vi "Select Controls 2.vi"(10 "All Controls[]":refnum<vi>[](array[refnum])=[refnum, refnum, refnum, refnum, refnum, refnum, refnum, refnum, refnum]) -> (0 "Create Accessors Folder 2":bool=TRUE, 1 "OK?":bool, 2 "Selection":i32[](array[numeric]), 3 "Operation":T1, 4 "Create Properties 2":bool, 5 "isDynamic?":bool)   [LabVIEW 2018, in "DVR Accessor Library.lvlib"]
uses:
  DVR Accessor Library.lvlib
  TypeDef/Accessor Type.ctl
panel:
  in  "Create Accessors Folder on HD":bool=TRUE
  in  "Type":T1=enum."Read And Write"
  in  "Scope":enum32{"Item 0", "Item 1"}(radio)
  in  "Create Properties":bool=TRUE
  in  "Cancel":bool
  in  "OK":bool
  in  "Data Members":string[](tree)
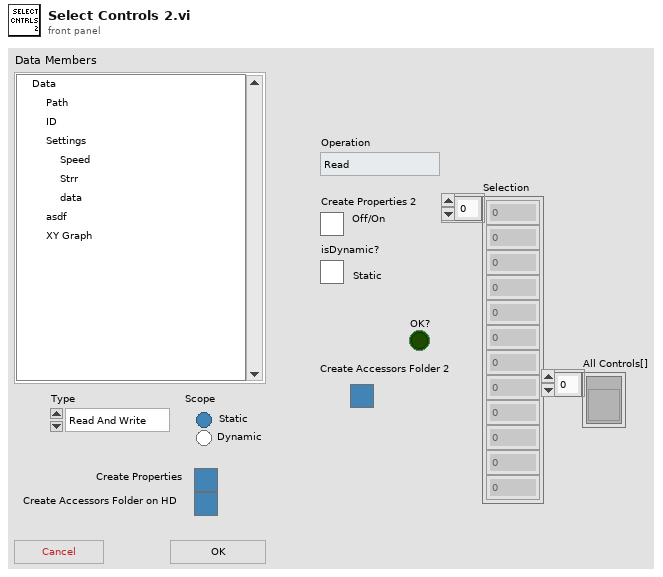
[diagram p1: front panel]
types:
  T1 = typedef "DVR Accessor Library.lvlib/Accessor Type.ctl" = enum16{"Read", "Read And Write", "Write"}
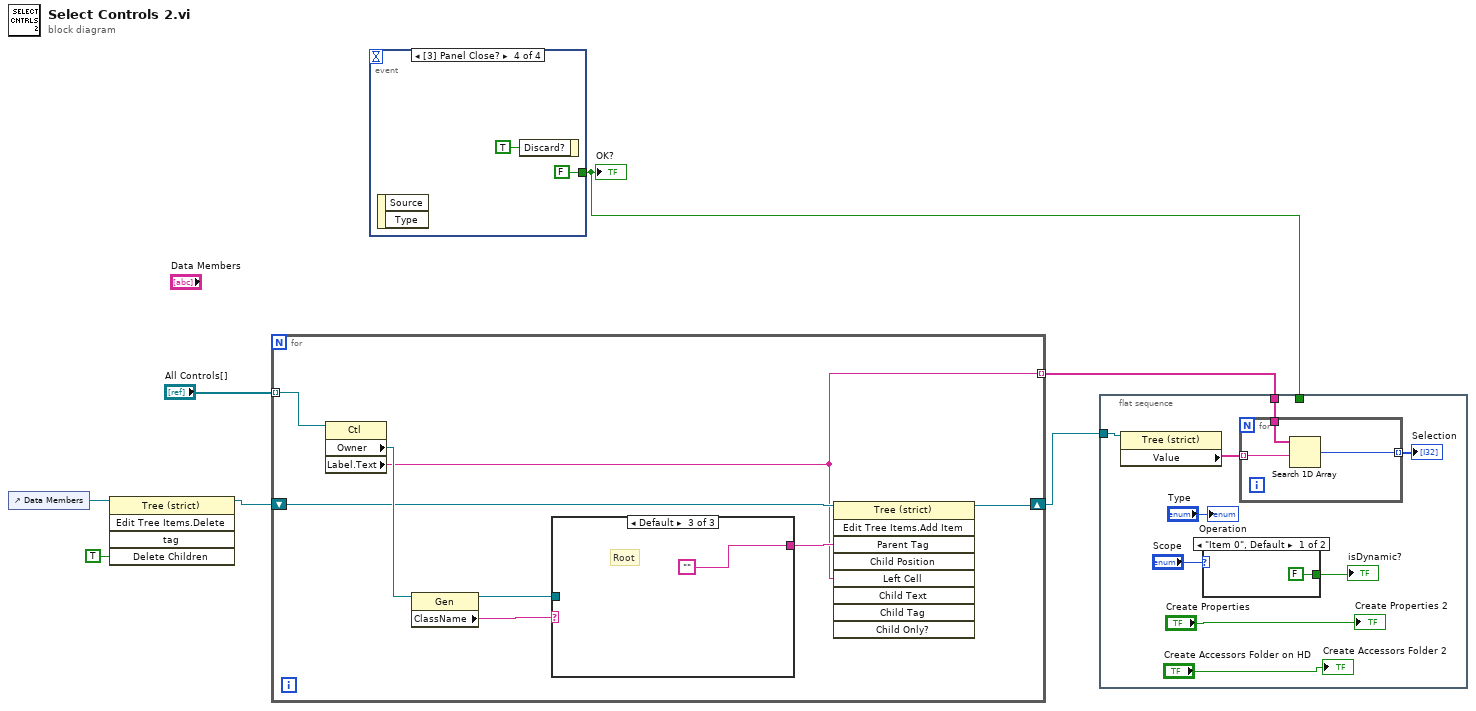
[diagram p0: block diagram]
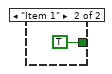
[diagram p2: hidden frame]
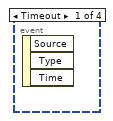
[diagram p3: hidden frame]
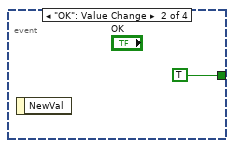
[diagram p4: hidden frame]
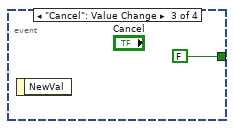
[diagram p5: hidden frame]
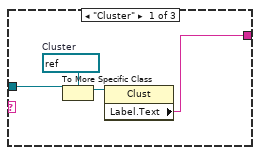
[diagram p6: hidden frame]
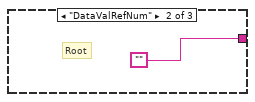
[diagram p7: hidden frame]
diagram:
  n1 = control-ref of="Data Members"() -> (w6:refnum<vi>)
  n2 = invoke class="Tree (strict)" method="Edit Tree Items.Delete"(reference=w6, "Delete Children"=TRUE ("Delete Children?")) -> (reference out=w5:refnum<vi>)  [unwired: 3 in, 4 out]
  n3 = for {
    tunnel: "All Controls[]" -> [w15] mode=indexing
    shift-right: [w9] -> w3
    shift-left: w5 -> [w13]
    tunnel: [w8] -> w2 mode=indexing
    n4 = property class="Ctl"(reference=w15) -> ("Owner"=w14:refnum<vi>, "Label.Text"=w8:string)  [unwired: 1 in, 2 out]
    n5 = property class="Gen"(reference=w14) -> (reference out=w10:refnum<vi>, "ClassName"=w12:string)  [unwired: 1 in, 1 out]
    n6 = case shown="Default" w12 {
      tunnel: [w16 "" ""] -> w11
      tunnel: w10 -> [w19 _ _]
      frame "Cluster" {
        w18 = refnum<vi> refnum  # Cluster
        n7 = To More Specific Class(target class=w18, reference=w19) -> (specific class reference=w17:refnum<vi>)  [unwired: 1 in, 1 out]
        n8 = property class="Clust"(reference=w17) -> ("Label.Text"=w16:string)  [unwired: 1 in, 2 out]
      }
      frame "DataValRefNum" {
        # "Root"
      }
      frame Default {
        # "Root"
      }
    }
    n9 = invoke on="Invoke Node" class="Tree (strict)" method="Edit Tree Items.Add Item"(reference=w13, "Parent Tag"=w11, "Left Cell"=w8) -> (reference out=w9:refnum<vi>)  [unwired: 6 in, 8 out]
  }
  n10 = event shown="[3] Panel Close?" {
    selector: _ -> [_ _ _ _]
    dyn-events: _ -> [_ _ _ _]
    timeout: _ -> [_ _ _ _]
    tunnel: [_ TRUE FALSE FALSE] -> w1
    event Timeout {
      n11 = event-data() -> ()  [unwired: 1 in, 3 out]
    }
    event "OK": Value Change {
      n12 = event-data() -> ()  [unwired: 1 in, 1 out]
    }
    event "Cancel": Value Change {
      n13 = event-data() -> ()  [unwired: 1 in, 1 out]
    }
    event Panel Close? {
      n14 = event-data() -> ()  [unwired: 1 in, 2 out]
      n15 = event-data("Discard?"=TRUE) -> ()  [unwired: 1 in, 1 out]
    }
  }
  "OK?" <- w1
  n16 = flat-sequence {
    tunnel: w3 -> [w28]
    tunnel: w2 -> [w27]
    tunnel: w1 -> [_]
    frame #0 {
      n17 = property on="Property Node" class="Tree (strict)"(reference=w28) -> ("Value"=w29:string[])  [unwired: 1 in, 2 out]
      n18 = case shown="\"Item 0\", Default" "Scope" {
        tunnel: [FALSE TRUE] -> w31
        frame "Item 0", Default {
        }
        frame "Item 1" {
        }
      }
      "isDynamic?" <- w31
      n19 = for {
        tunnel: w29 -> [w37] mode=indexing
        tunnel: [w36] -> w30 mode=indexing
        tunnel: w27 -> [w35]
        n20 = Search 1D Array(1D array=w35, element=w37) -> (index of element=w36:i32)  [unwired: 1 in]
      }
      "Selection" <- w30
      "Operation" <- "Type"
      "Create Properties 2" <- "Create Properties"
      "Create Accessors Folder 2" <- "Create Accessors Folder on HD"
    }
  }
